vi "Servo MSMT Set RF WFM Parameters.vi"(8 "error in (no error)":errorcluster, 10 "Step In":refnum<k7>, 11 "Servo MSMT in":refnum<class "Servo MSMT.lvclass">) -> (0 "error out":errorcluster, 2 "Step Out":refnum<k7>, 3 "Servo MSMT out":refnum<class "Servo MSMT.lvclass">)   [LabVIEW 2014, in "Servo MSMT.lvclass"]
uses:
  Servo MSMT.lvclass
  Measurement Interface/Measurement Interface.lvlibp/Private Methods/Measurement Parameters/Read Measurement Parameters.vi
  Includes/String Database/String Database.lvlibp/String Database.lvclass
  QPA Measurement/QPA Measurement.lvlibp/Sequence Automation/Classes/QPA Measurement/QPA Measurement.lvclass
  TestStand API Tools/Step Actions/TSAT Step Actions.lvlib
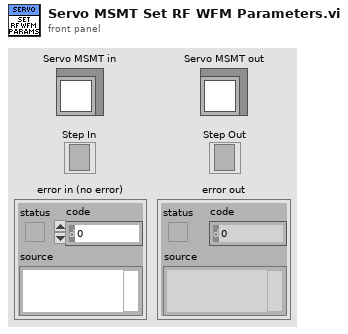
[diagram p1: front panel]
types:
  T1 = typedef "QPA Measurement.lvlibp/QPA MSMT Waveform Manager.lvclass/RF Waveform.ctl" = cluster{"Name":string, "Path":path, "Headroom":dbl, "Burst Length":dbl}
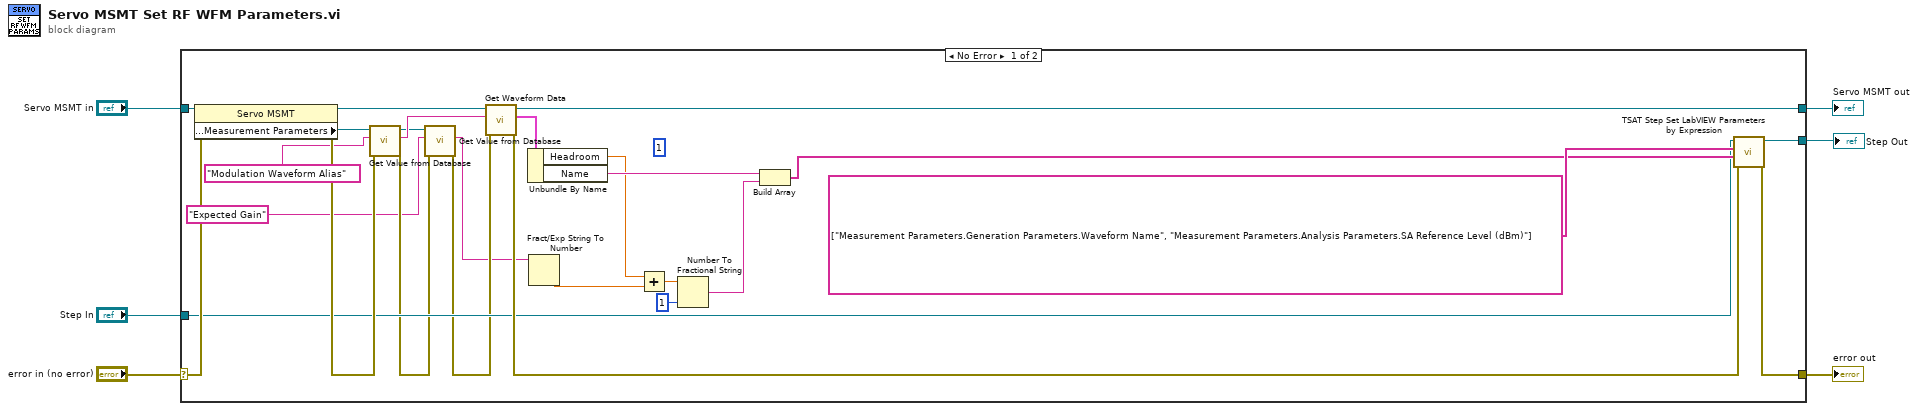
[diagram p0: block diagram]
diagram:
  n1 = case shown="No Error" "error in (no error)" {
    selector: "error in (no error)" -> [w32 w35]
    tunnel: [w28 w35] -> w5
    tunnel: [w22 w34] -> w3
    tunnel: "Servo MSMT in" -> [w27 w34]
    tunnel: [w19 w33] -> w2
    tunnel: "Step In" -> [w18 w33]
    frame No Error {
      (unwired) i16 1 ("precision (6)")
      n2 = property class="Servo MSMT"(reference=w27, error in=w32) -> (reference out=w26:refnum<class "Servo MSMT.lvclass">, error out=w24:errorcluster, "Protected Methods:Measurement Parameters"=w25:refnum<class "String Database.lvclass">)
      n3 = call "Get Value from Database.vi"("error in (no error)"=w24, "Entry Name"="Modulation Waveform Alias", "Message in"=w25) -> ("error out"=w15:errorcluster, "Entry Value"=w17:string, "Message out"=w16:refnum<class "String Database.lvclass">)  [unwired: 5 in, 1 out]
      n4 = call "Get Value from Database.vi"("error in (no error)"=w15, "Entry Name"="Expected Gain", "Message in"=w16) -> ("error out"=w14:errorcluster, "Entry Value"=w12:string)  [unwired: 5 in, 2 out]
      n5 = call "Get Waveform Data.vi"("error in (no error)"=w14, "Waveform to Retrieve"=w17, "QPA Measurement in"=w26) -> ("error out"=w31:errorcluster, "RF Waveform"=w30:T1, "QPA Measurement out"=w22:refnum<class "Servo MSMT.lvclass">)  [unwired: 6 in]
      n6 = Unbundle By Name(w30) -> ("Headroom"=w11:dbl, "Name"=w29:string)
      n7 = Fract/Exp String To Number(string=w12) -> (number=w10:dbl)  [unwired: 3 in, 1 out]
      n8 = Add(x=w11, y=w10) -> (x+y=w9:dbl)
      n9 = Number To Fractional String(number=w9, precision (6)=i16 1) -> (F-format string=w8:string)  [unwired: 2 in]
      n10 = Build Array(w29, w8) -> (w20:string[])
      n11 = call "TSAT Step Set LabVIEW Parameters by Expression.vi"("Error In"=w31, "Value Expressions"=w20, "Parameters to Set"=string[] ["Measurement Parameters.Generation Parameters.Waveform Name", "Measurement Parameters.Analysis Parameters.SA Reference Level (dBm)"], "Step In"=w18) -> ("Error Out"=w28:errorcluster, "Step Out"=w19:refnum<k7>)  [unwired: 6 in]
    }
    frame Error {
    }
  }
  "error out" <- w5
  "Servo MSMT out" <- w3
  "Step Out" <- w2
